vi "Open.vi"(0 "AD2 I2C In":refnum<class "AD2 I2C.lvclass">, 5 "WaveForms Session In":T1, 7 "Power Supply Voltage":dbl=3.3 format="%#_13g", 9 "hz":dbl=100000.0 format="%#_13g", 11 "Error In":errorcluster, 12 "SCL idxChannel":i32, 13 "SDA idxChannel":i32=1) -> (4 "AD2 I2C Out":refnum<class "AD2 I2C.lvclass">, 15 "Error Out":errorcluster)   [LabVIEW 2020, in "lv_i2c_ad2.lvlib" / "AD2 I2C.lvclass"]
uses:
  AD2 I2C.lvclass
  lv_waveforms_toolkit/WFT Session.ctl
  AD2 I2C.lvclass/AD2 I2C.ctl
  lv_waveforms_toolkit/lv_waveforms_toolkit.lvlib
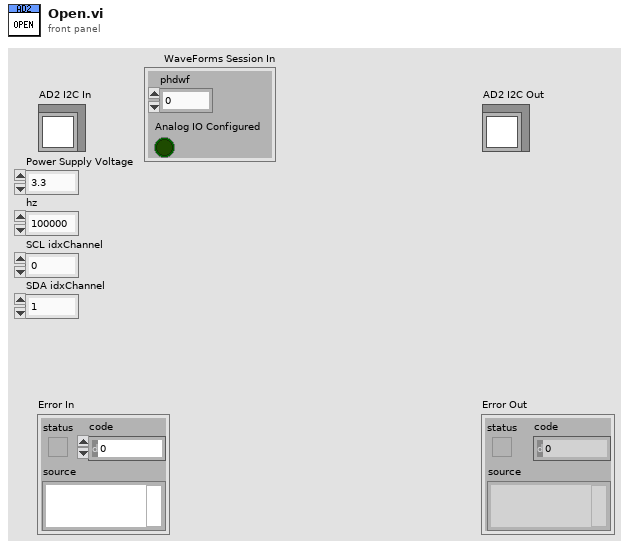
[diagram p1: front panel]
types:
  T1 = typedef "lv_waveforms_toolkit.lvlib/WFT Session.ctl" = cluster{"phdwf":i32, "Analog IO Configured":bool}
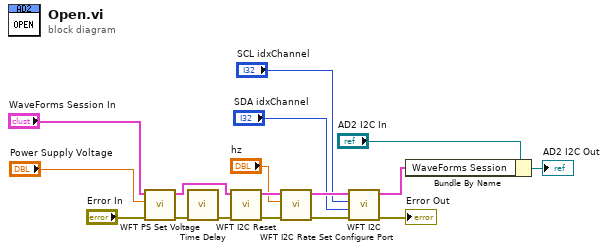
[diagram p0: block diagram]
diagram:
  n1 = call "WFT PS Set Voltage.vi"("Error In"="Error In", "Voltage"="Power Supply Voltage", "WaveForms Session In"="WaveForms Session In") -> ("Error Out"=w16:errorcluster, "WaveForms Session Out"=w11:T1)  [unwired: 7 in]
  n2 = call "Time Delay"("error in (no error)"=w16) -> ("error out"=w9:errorcluster)  [unwired: 10 in]
  n3 = call "WFT I2C Reset.vi"("Error In"=w9, "WaveForms Session In"=w11) -> ("Error Out"=w8:errorcluster, "WaveForms Session Out"=w10:T1)  [unwired: 7 in, 1 out]
  n4 = call "WFT I2C Rate Set.vi"("Error In"=w8, "hz"="hz", "WaveForms Session In"=w10) -> ("Error Out"=w14:errorcluster, "WaveForms Session Out"=w15:T1)  [unwired: 6 in, 1 out]
  n5 = call "WFT I2C Configure Port.vi"("Error In"=w14, "SDA idxChannel"="SDA idxChannel", "SCL idxChannel"="SCL idxChannel", "WaveForms Session In"=w15) -> ("Error Out"=→"Error Out":errorcluster, "WaveForms Session Out"=w3:T1)  [unwired: 4 in, 2 out]
  n6 = Bundle By Name(cluster="AD2 I2C In", "WaveForms Session"=w3) -> (→"AD2 I2C Out":refnum<class "AD2 I2C.lvclass">)
